vi "Module API.vi"(8 "error in (no error)":errorcluster, 11 "OtherModule in":refnum<class "OtherModule.lvclass">) -> (0 "error out":errorcluster, 2 "API":refnum<class "API.lvclass">, 3 "OtherModule out":refnum<class "OtherModule.lvclass">)   [LabVIEW 2020]
uses:
  OtherModule.lvclass/OtherModule.ctl
  Volatus/API/API.lvclass
  OtherModule.lvclass
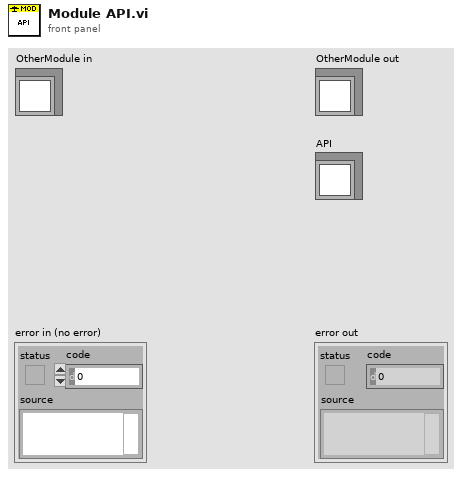
[diagram p1: front panel]
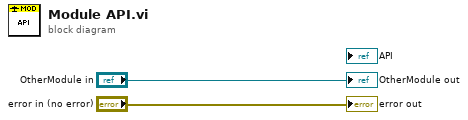
[diagram p0: block diagram]
diagram:
  "error out" <- "error in (no error)"
  "OtherModule out" <- "OtherModule in"
